vi "Write loopTimer.vi"(8 "error in (no error)":errorcluster, 10 "ILoopTimer.lvclass":refnum<class "ILoopTimer.lvclass">, 11 "WindowsTarget in":refnum<class "cRIOScanModeTarget.lvclass">) -> (0 "error out":errorcluster, 3 "WindowsTarget out":refnum<class "cRIOScanModeTarget.lvclass">)   [LabVIEW 2012, in "cRIOScanModeTarget.lvclass"]
uses:
  cRIOScanModeTarget.lvclass
  <userlib>/Common/ComponentModel/ComponentModelRT/LoopTimer/ILoopTimer/ILoopTimer.lvclass
  cRIOScanModeTarget.lvclass/cRIOScanModeTarget.ctl
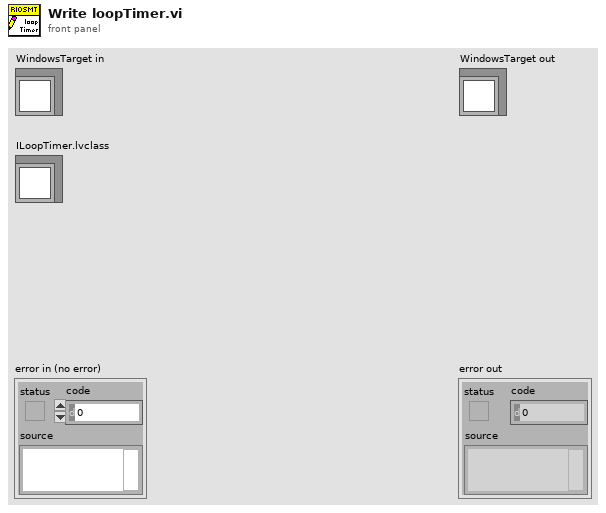
[diagram p1: front panel]
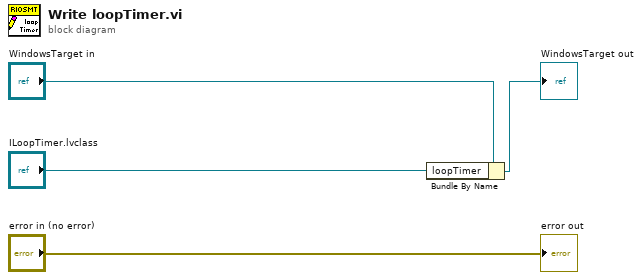
[diagram p0: block diagram]
diagram:
  n1 = Bundle By Name(cluster="WindowsTarget in", "loopTimer"="ILoopTimer.lvclass") -> (→"WindowsTarget out":refnum<class "cRIOScanModeTarget.lvclass">)
  "error out" <- "error in (no error)"
